vi "ProcessReading.vi"(11 "file path (dialog if empty)":path) -> (2 "Y":dbl, 3 "X":dbl)   [LabVIEW 2016]
uses:
  <vilib>/Utility/file.llb/Read Delimited Spreadsheet (DBL).vi
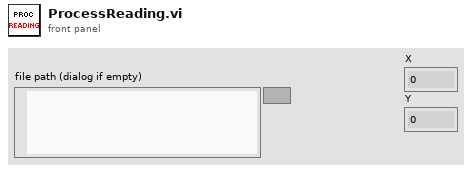
[diagram p1: front panel]
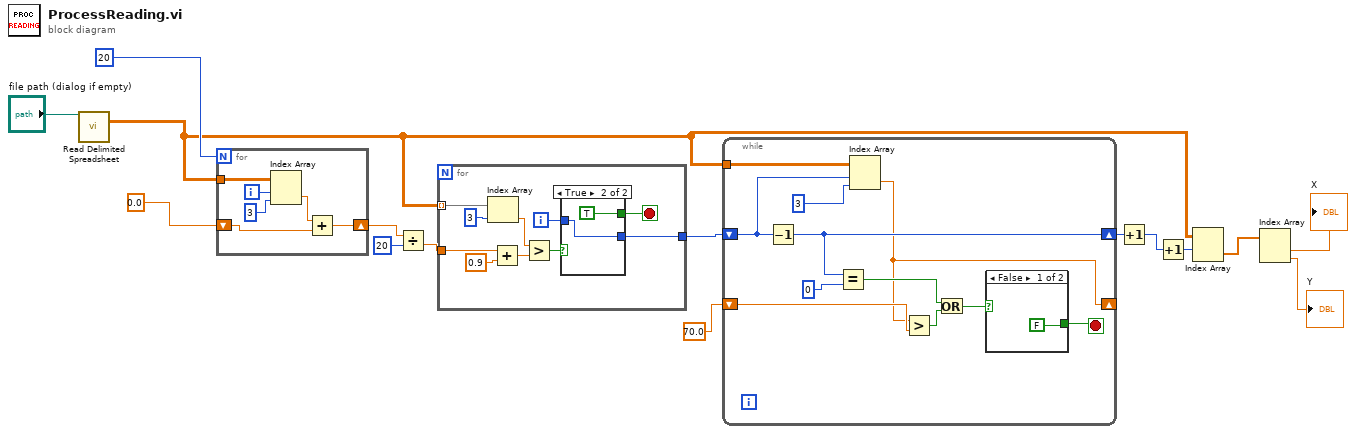
[diagram p0: block diagram]
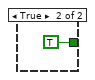
[diagram p2: hidden frame]
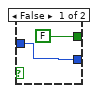
[diagram p3: hidden frame]
diagram:
  n1 = call-poly <vilib>:"Read Delimited Spreadsheet.vi"("file path (dialog if empty)"="file path (dialog if empty)") -> ("all rows"=w7:dbl[][])  [unwired: 9 in, 5 out]
  n2 = for {
    N: 20 -> [_]
    tunnel: w7 -> [w21]
    shift-right: [w16] -> w12
    shift-left: 0.0 -> [w17]
    i -> [w20]
    n3 = Index Array(array=w21, index (row)=w20, index (col)=3) -> (element=w18:dbl)
    n4 = Add(x=w18, y=w17) -> (x+y=w16:dbl)
  }
  n5 = Divide(x=w12, y=20) -> (x/y=w10:dbl)
  n6 = for {
    tunnel: w7 -> [w31] mode=indexing
    tunnel: w10 -> [w28]
    tunnel: [w22] -> w6
    i -> [w23]
    stop <- w24 stop-if-true
    n7 = Index Array(array=w31, index=3) -> (element=w29:dbl)
    n8 = Add(x=w28, y=0.9) -> (x+y=w26:dbl)
    n9 = Greater?(x=w29, y=w26) -> (0:w25:bool)
    n10 = case shown="True" w25 {
      tunnel: [FALSE TRUE] -> w24
      tunnel: [w32 w34] -> w22
      tunnel: w23 -> [w32 w34]
      frame False {
      }
      frame True {
      }
    }
  }
  n11 = while {
    shift-right: [w41] -> w8
    shift-left: w6 -> [w45]
    tunnel: w7 -> [w46]
    shift-right: [w36] -> _
    shift-left: 70.0 -> [w43]
    stop <- w42 stop-if-true
    n12 = Decrement(x=w45) -> (x-1=w41:i32)
    n13 = Equal?(x=w41, y=0) -> (x = y?=w39:bool)
    n14 = Index Array(array=w46, index (row)=w45, index (col)=3) -> (element=w36:dbl)
    n15 = Greater?(x=w36, y=w43) -> (0:w38:bool)
    n16 = Or(x=w39, y=w38) -> (x .or. y?=w37:bool)
    n17 = case shown="False" w37 {
      tunnel: [FALSE TRUE] -> w42
      frame False {
      }
      frame True {
      }
    }
  }
  n18 = Increment(x=w8) -> (x+1=w5:i32)
  n19 = Increment(x=w5) -> (x+1=w4:i32)
  n20 = Index Array(array=w7, index (row)=w4) -> (element=w3:dbl[])  [unwired: 1 in]
  n21 = Index Array(array=w3) -> (element #1=→"X":dbl, element #2=→"Y":dbl)  [unwired: 2 in]
